vi "Focus_vs_Field.vi"(7 "Dist (Field)":dbl, 8 "a3":dbl format="%.3e", 9 "a2":dbl format="%.3e", 10 "a1":dbl format="%.3e", 11 "a0":dbl) -> (0 "Correction":i32, 3 "Focus (table)":dbl)   [LabVIEW 2011]
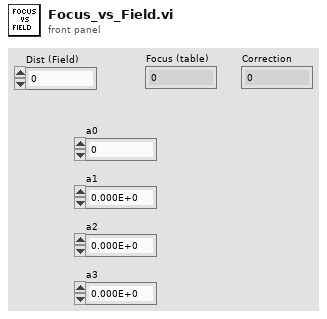
[diagram p1: front panel]
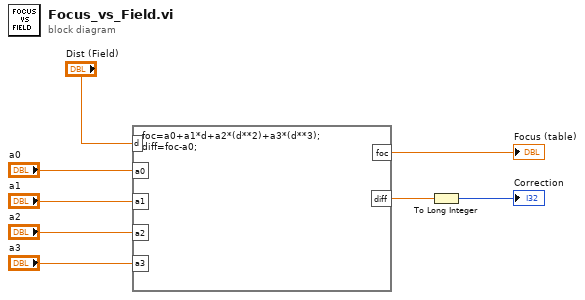
[diagram p0: block diagram]
diagram:
  n1 = formula code="foc=a0+a1*d+a2*(d**2)+a3*(d**3);\ndiff=foc-a0;"("a0"="a0", "a1"="a1", "a2"="a2", "a3"="a3", "d"="Dist (Field)") -> ("foc"=→"Focus (table)":dbl, "diff"=w2:dbl)
  n2 = To Long Integer(number=w2) -> (32bit integer=→"Correction":i32)
